vi "load_specification_file.vi"(9 "LUA Specification File":path, 10 "Parameters Tree":refnum<vi>, 11 "# Lines":refnum<vi>) -> (2 "Spec File Loaded":bool)   [LabVIEW 2019]
uses:
  lib/libSpecValiReader.so
  lib/libSimulationControl/libSimulationControl.lvlib
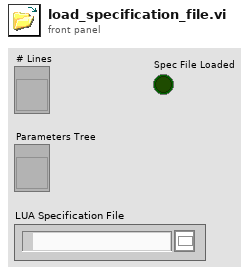
[diagram p1: front panel]
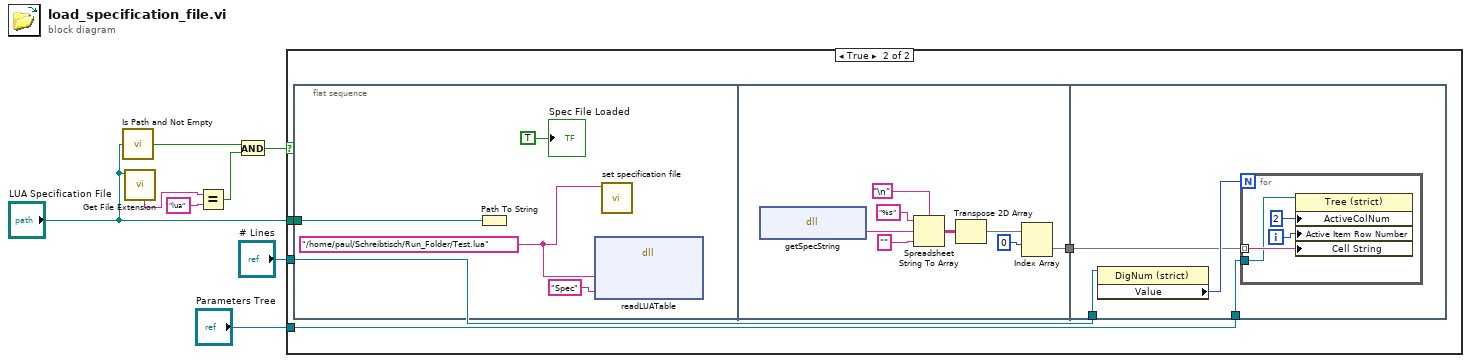
[diagram p0: block diagram]
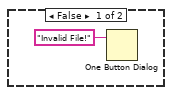
[diagram p2: hidden frame]
diagram:
  n1 = call <vilib>:"Is Path and Not Empty.vi"("path"="LUA Specification File") -> ("Is Path and Not Empty?"=w4:bool)  [unwired: 4 in]
  n2 = call <vilib>:"Get File Extension.vi"("file"="LUA Specification File") -> ("unmodified file extension"=w6:string)  [unwired: 6 in, 4 out]
  n3 = Equal?(x=w6, y="lua") -> (x = y?=w3:bool)
  n4 = And(x=w4, y=w3) -> (x .and. y?=w1:bool)
  n5 = case shown="True" w1 {
    tunnel: "Parameters Tree" -> [_ w12]
    tunnel: "# Lines" -> [_ w11]
    tunnel: "LUA Specification File" -> [_ w10]
    frame False {
      n6 = One Button Dialog(message="Invalid File!") -> ()  [unwired: 1 in, 1 out]
    }
    frame True {
      n7 = flat-sequence {
        tunnel: w10 -> [w16]
        tunnel: [w19] -> w13
        tunnel: w13 -> [w28]
        tunnel: w12 -> [w27]
        tunnel: w11 -> [w26]
        frame #0 {
          w14 = "/home/paul/Schreibtisch/Run_Folder/Test.lua" ("filename")
          n8 = Path To String(path=w16) -> ()  [unwired: 1 out]
          n9 = dll-call lib="home/paul/Schreibtisch/Biogas_plant_setup/lib/libSpecValiReader.so" fn="readLUATable"("filename"=w14, "vali_or_spec"="Spec" ("spec_filename")) -> ()  [unwired: 6 in, 2 out]
          n10 = call "set specification file.vi"("spec_file"=w14) -> ()  [unwired: 10 in, 1 out]
          "Spec File Loaded" <- TRUE ("Value")
        }
        frame #1 {
          n11 = dll-call lib="home/paul/Schreibtisch/Biogas_plant_setup/lib/libSpecValiReader.so" fn="getSpecString"() -> ("return type"=w23:string)  [unwired: 3 in, 2 out]
          n12 = Spreadsheet String To Array(delimiter (Tab)="\n", format string="%s", spreadsheet string=w23, array type (2D Dbl)="") -> (array=w24:string[][])
          n13 = Transpose 2D Array(2D array=w24) -> (transposed array=w25:string[][])
          n14 = Index Array(array=w25, index (row)=0) -> (element=w19:string[])  [unwired: 1 in]
        }
        frame #2 {
          n15 = property class="DigNum (strict)"(reference=w26) -> ("Value"=w29:i32)  [unwired: 1 in, 2 out]
          n16 = for {
            N: w29 -> [_]
            tunnel: w28 -> [w31] mode=indexing
            tunnel: w27 -> [w30]
            i -> [w32]
            n17 = property on="Property Node" class="Tree (strict)"(reference=w30, "ActiveColNum"=2 ("Active Cell:Active Column Number"), "Active Item Row Number"=w32, "Cell String"=w31) -> ()  [unwired: 1 in, 2 out]
          }
        }
      }
    }
  }
